vi "SR Status Filter(SubVI).vi"(7 "Filter Parameters":string[](array[string]), 11 "SR Data In":T1[](array[typedef])) -> (3 "SR DataOut":T1[](array[typedef]), 6 "Filtered Out SRs":T1[](array[typedef]))   [LabVIEW 2017, in "DS_Lib.lvlib" / "SRReportParser.lvlib"]
uses:
  Modules/Private Controls/Data Raw.ctl
  SRReportParser.lvlib
  Modules/Data Operations.lvlib
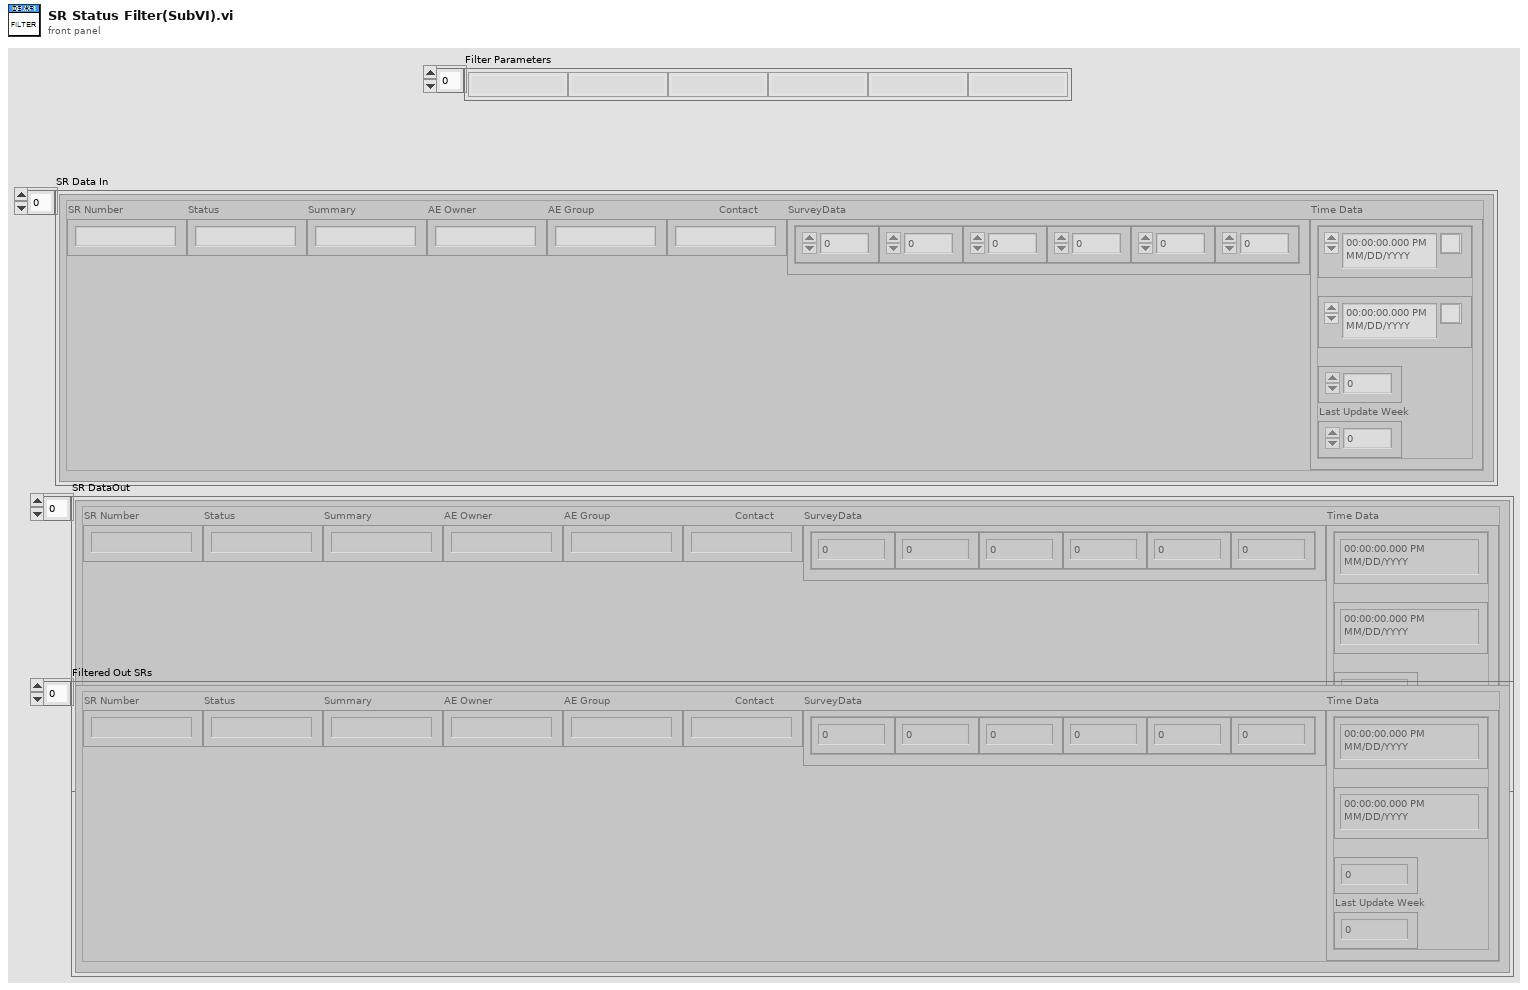
[diagram p1: front panel]
types:
  T1 = typedef "Data Operations.lvlib/Data Raw.ctl" = cluster{"SR Number":string, "Status":string, "Summary":string, "AE Owner":string, "AE Group":string, "Contact":string, "SurveyData":cluster{"Resolution Time":dbl, "Total Satisfaction":dbl, "Response Time":dbl, "Courtesy":dbl, "Problem Solved":dbl, "Level of effort":dbl}, "Time Data":cluster{"Last Update Date":timestamp, "Creation Date":timestamp, "Creation week":u8, "Last Update Week":u8}}
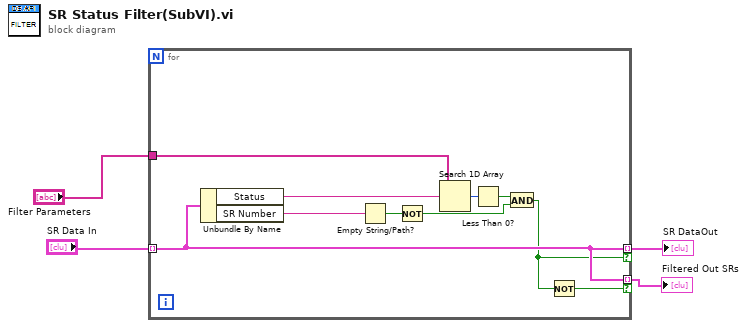
[diagram p0: block diagram]
diagram:
  n1 = for {
    tunnel: "SR Data In" -> [w12] mode=indexing
    tunnel: "Filter Parameters" -> [w14]
    tunnel: [w12] -> w3 mode=indexing if=w5
    tunnel: [w12] -> w1 mode=indexing if=w11
    n2 = Unbundle By Name(w12) -> ("Status"=w8:string, "SR Number"=w9:string)
    n3 = Empty String/Path?(string/path=w9) -> (empty?=w10:bool)
    n4 = Not(x=w10) -> (.not. x?=w6:bool)
    n5 = Search 1D Array(1D array=w14, element=w8) -> (index of element=w13:i32)  [unwired: 1 in]
    n6 = Less Than 0?(x=w13) -> (x < 0?=w7:bool)
    n7 = And(x=w7, y=w6) -> (x .and. y?=w5:bool)
    n8 = Not(x=w5) -> (.not. x?=w11:bool)
  }
  "SR DataOut" <- w3
  "Filtered Out SRs" <- w1
